vi "JLINKARM ReadFile.vi"(8 "error in (no error)":errorcluster, 11 "Path In":path) -> (0 "error out":errorcluster, 2 "Data":T1[](array[typedef]) {"Data" format="%02x"; "Addr" format="%08x"}, 3 "Path Out":path, 4 "ReadFileTime(ms)":u32, 5 "DecodeTime(ms)":u32)   [LabVIEW 2016]
uses:
  <userlib>/LV-JLinkARM/App/JLINKARM AllDataType.ctl
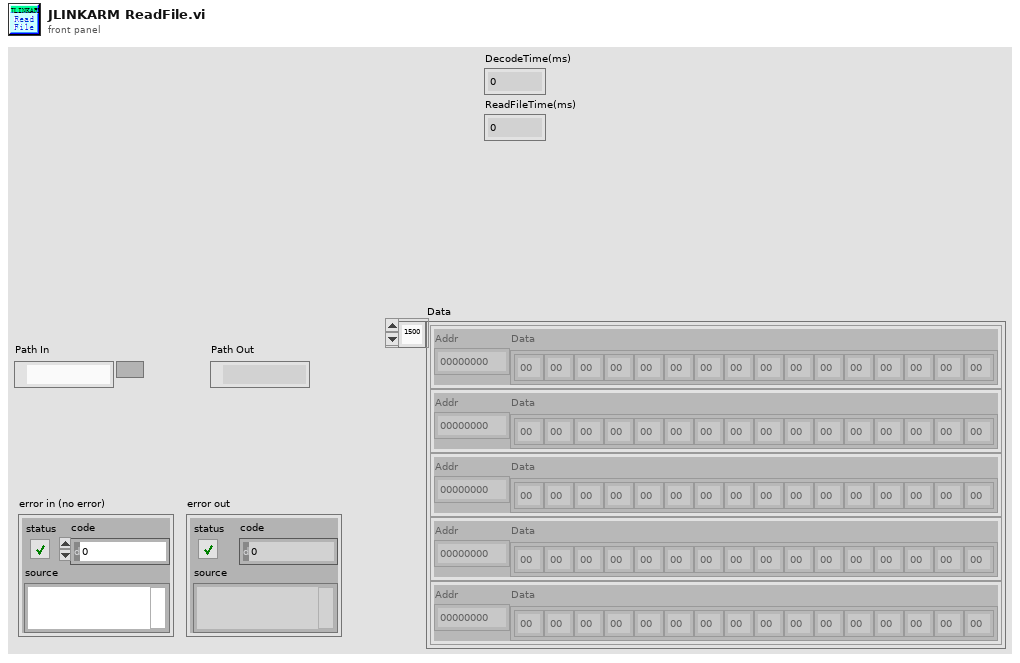
[diagram p1: front panel]
types:
  T1 = typedef "JLINKARM AllDataType.ctl" = cluster{"Addr":u32, "Data":u8[]}
  T2 = typedef "JLinkARM LineHexDataType.ctl" = cluster{"Len":u8, "Addr":u16, "Type":T3, "Data":u8[], "CRC":u8}
  T3 = typedef "JLINKARM DataType.ctl" = enum16{"Data", "EndofFile", "ExtSegAdd", "StartSegAddr", "ExtLinearAddr", "StartLinearAddr"}
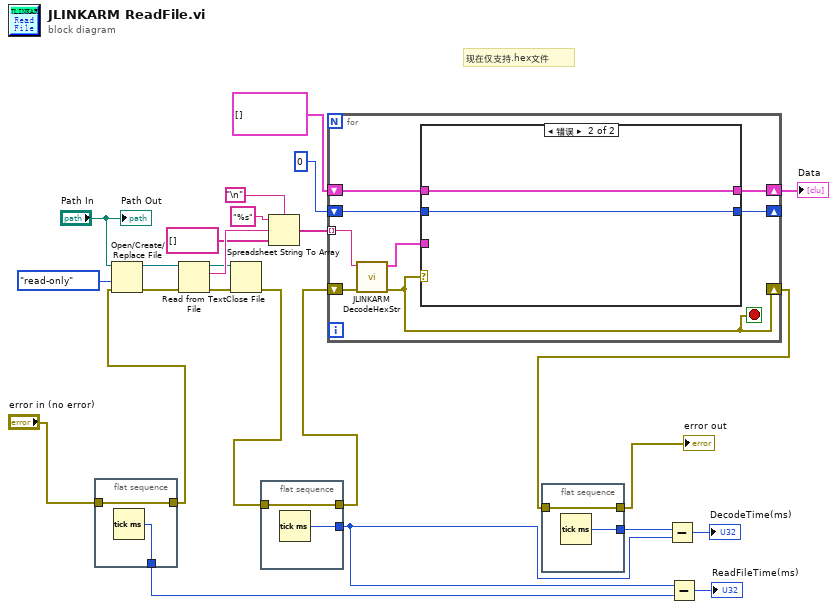
[diagram p0: block diagram]
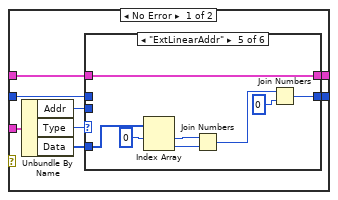
[diagram p2: hidden frame]
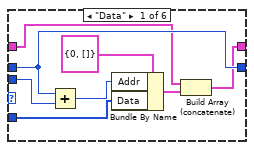
[diagram p3: hidden frame]
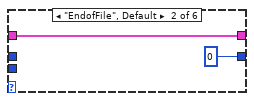
[diagram p4: hidden frame]
diagram:
  # "现在仅支持.hex文件"
  n1 = flat-sequence {
    tunnel: [w27] -> w11
    tunnel: "error in (no error)" -> [w27]
    tunnel: [w26] -> w4
    frame #0 {
      n2 = Tick Count (ms)() -> (millisecond timer value=w26:u32)
    }
  }
  n3 = Open/Create/Replace File(file path (use dialog)="Path In", error in=w11, access (0:read/write)=enum16{"read/write", "read-only", "write-only"}."read-only") -> (refnum out=w24:refnum<file>, error out=w23:errorcluster)  [unwired: 3 in, 1 out]
  n4 = Read from Text File(file (use dialog)=w24, error in=w23) -> (refnum out=w18:refnum<file>, text=w22:string, error out=w19:errorcluster)  [unwired: 2 in, 1 out]
  n5 = Close File(refnum=w18, error in=w19) -> (error out=w1:errorcluster)  [unwired: 1 out]
  n6 = flat-sequence {
    tunnel: [w29] -> w9
    tunnel: w1 -> [w29]
    tunnel: [w28] -> w5
    frame #0 {
      n7 = Tick Count (ms)() -> (millisecond timer value=w28:u32)
    }
  }
  n8 = Spreadsheet String To Array(delimiter (Tab)="\n", format string="%s", spreadsheet string=w22, array type (2D Dbl)=string[] []) -> (array=w15:string[])
  n9 = for {
    shift-right: [w30] -> w8
    shift-left: w9 -> [w37]
    tunnel: w15 -> [w36] mode=indexing
    shift-right: [w31] -> w12
    shift-left: T1[] [] -> [w32]
    shift-right: [w34] -> _
    shift-left: u32 0 -> [w33]
    stop <- w30 stop-if-true
    n10 = call <userlib>:"JLINKARM DecodeHexStr.vi"("错误输入（无错误）"=w37, "HexStr"=w36) -> ("错误输出"=w30:errorcluster, "LineHexData"=w35:T2)  [unwired: 8 in]
    n11 = case shown="错误" w30 {
      tunnel: w35 -> [w45 _]
      tunnel: [w42 w70] -> w34
      tunnel: w33 -> [w41 w70]
      tunnel: w32 -> [w39 w71]
      tunnel: [w38 w71] -> w31
      frame No Error {
        n12 = Unbundle By Name(w45) -> ("Addr"=w43:u16, "Type"=w44:T3, "Data"=w40:u8[])
        n13 = case shown="\"ExtLinearAddr\"" w44 {
          tunnel: w43 -> [w52 _ _ _ _ _]
          tunnel: [w53 u32 0 w57 w59 w60 w69] -> w42
          tunnel: w41 -> [w53 _ w57 w59 _ w69]
          tunnel: w40 -> [w50 _ _ _ w66 _]
          tunnel: w39 -> [w48 w54 w56 w58 w67 w68]
          tunnel: [w46 w54 w56 w58 w67 w68] -> w38
          frame "Data" {
            n14 = Add(x=w53, y=w52) -> (x+y=w51:u32)
            n15 = Bundle By Name(cluster=T1 {"Addr"=0, "Data"=[]} ("AllData"), "Addr"=w51, "Data"=w50) -> (w47:T1)
            n16 = Build Array (concatenate)(w48, w47) -> (w46:T1[])
          }
          frame "EndofFile", Default {
          }
          frame "ExtSegAdd" {
          }
          frame "StartSegAddr" {
          }
          frame "ExtLinearAddr" {
            n17 = Index Array(array=w66, index #1=0 ("索引")) -> (element #1=w64:u8, element #2=w63:u8)  [unwired: 1 in]
            n18 = Join Numbers(hi=w64, lo=w63) -> ((hi.lo)=w62:u16)
            n19 = Join Numbers(hi=w62, lo=u16 0) -> ((hi.lo)=w60:u32)
          }
          frame "StartLinearAddr" {
          }
        }
      }
      frame Error {
      }
    }
  }
  "Data" <- w12
  n20 = flat-sequence {
    tunnel: [w73] -> w7
    tunnel: w8 -> [w73]
    tunnel: [w72] -> w6
    frame #0 {
      n21 = Tick Count (ms)() -> (millisecond timer value=w72:u32)
    }
  }
  n22 = Subtract(x=w6, y=w5) -> (x-y=→"DecodeTime(ms)":u32)
  n23 = Subtract(x=w5, y=w4) -> (x-y=→"ReadFileTime(ms)":u32)
  "error out" <- w7
  "Path Out" <- "Path In"
